vi "Move Needle Impl.vi"(8 "error in (no error)":errorcluster, 10 "Needle Position":T1, 11 "Alltesta Autosampler in":refnum<class "Alltesta Autosampler.lvclass">) -> (0 "error out":errorcluster, 3 "Alltesta Autosampler out":refnum<class "Alltesta Autosampler.lvclass">)   [LabVIEW 2023, in "Alltesta Autosampler.lvlib" / "Alltesta Autosampler.lvclass"]
uses:
  Alltesta Autosampler.lvclass
  Autosampler/Autosampler Needle Position.ctl
  Alltesta Autosampler.lvclass/Alltesta Autosampler.ctl
  Alltesta Autosampler.lvlib
  Autosampler/Autosampler.lvlib
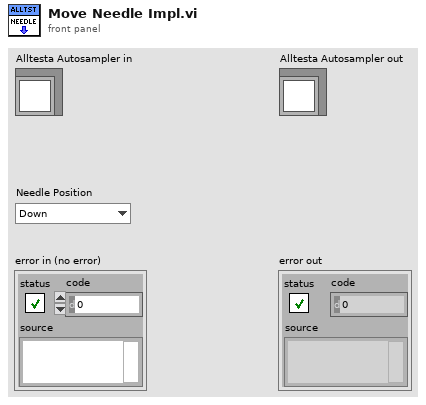
[diagram p1: front panel]
types:
  T1 = typedef "Autosampler.lvlib/Autosampler Needle Position.ctl" = enum16{"Down", "Up"}
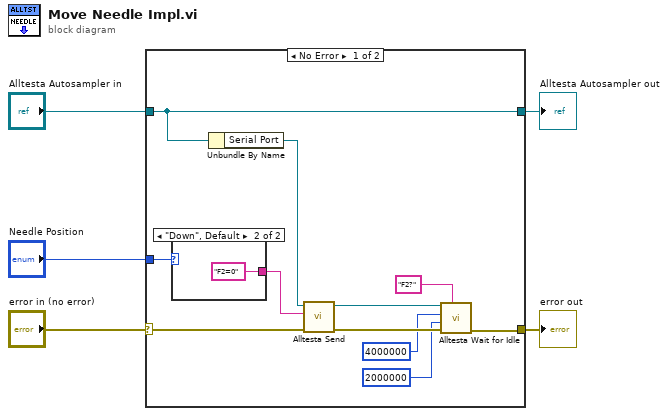
[diagram p0: block diagram]
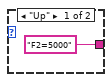
[diagram p2: hidden frame]
diagram:
  n1 = case shown="No Error" "error in (no error)" {
    selector: "error in (no error)" -> [w16 w19]
    tunnel: [w9 w19] -> w4
    tunnel: "Alltesta Autosampler in" -> [w13 w20]
    tunnel: [w13 w20] -> w2
    tunnel: "Needle Position" -> [w15 _]
    frame No Error {
      n2 = case shown="\"Down\", Default" w15 {
        tunnel: ["F2=5000" ("Raise needle") "F2=0" ("Raise needle")] -> w14
        frame "Up" {
        }
        frame "Down", Default {
        }
      }
      n3 = Unbundle By Name(w13) -> ("Serial Port"=w12:refnum<visa-resource-name>)
      n4 = call "Alltesta Send.vi"("error in (no error)"=w16, "Command"=w14, "Serial Port in"=w12) -> ("error out"=w11:errorcluster, "Serial Port out"=w10:refnum<visa-resource-name>)  [unwired: 6 in, 1 out]
      n5 = call "Alltesta Wait for Idle.vi"("Poll Command"="F2?" ("format string"), "error in (no error)"=w11, "Lower Bound"=2000000, "Upper Bound"=4000000, "Serial Port in"=w10) -> ("error out"=w9:errorcluster)  [unwired: 5 in, 1 out]
    }
    frame Error {
    }
  }
  "error out" <- w4
  "Alltesta Autosampler out" <- w2
